vi "General Histogram PtByPt.vi"(0 "x":dbl format="%0.2f", 1 "max":dbl format="%0.2f", 3 "initialize":bool, 5 "Bins":T2(array[cluster]) {"upper" format="%0.2f"; "lower" format="%0.2f"}, 9 "inclusion":enum16{"lower", "upper"}(ring), 11 "sample length":i32=100, 12 "min":dbl format="%0.2f", 14 "# bins":i32) -> (4 "Histogram Graph":T1(graph), 6 "Histogram":i32[](array[numeric]), 8 "Axis":dbl[](array[numeric]), 10 "# outside":cluster{"total":i32, "above":i32, "below":i32}, 15 "error":i32)   [LabVIEW 2020, in "NI_PtbyPt.lvlib"]
doc: "Finds the discrete histogram of the set of input data points specified by <B>sample length</B> based on the given bin specifications."
uses:
  <vilib>/ptbypt/NI_PtbyPt.lvlib
  <vilib>/Analysis/NI_AALPro.lvlib
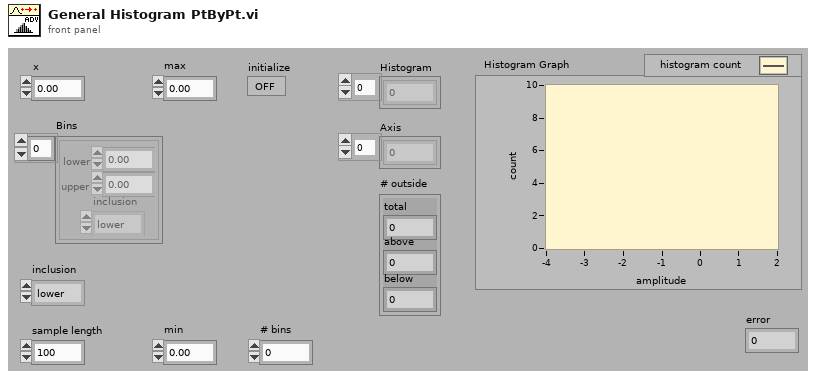
[diagram p1: front panel]
types:
  T1 = cluster{"X Values":dbl[], "Histogram: h(x)":i32[]}
  T2 = cluster{"lower":dbl, "upper":dbl, "inclusion":enum32{"lower", "upper", "both", "neither"}}[]
  T3 = cluster{"lower":dbl, "upper":dbl, "inclusion":u32}[]
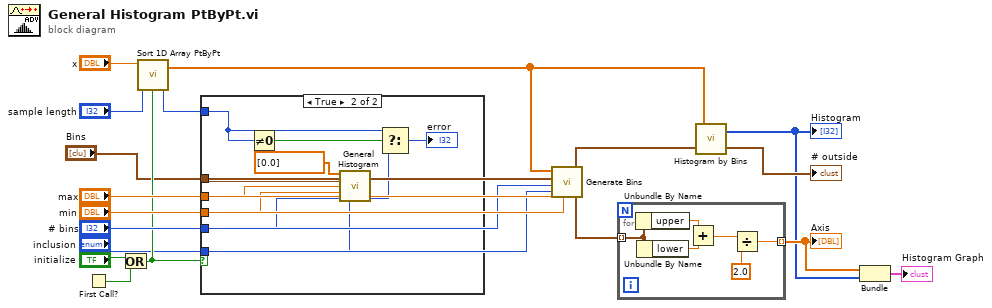
[diagram p0: block diagram]
diagram:
  n1 = First Call?() -> (First Call?: T/F=w7:bool)
  n2 = Or(x="initialize", y=w7) -> (x .or. y?=w9:bool)
  n3 = call <vilib>:"Sort 1D Array PtByPt.vi"("initialize"=w9, "sample length"="sample length", "input data point"="x") -> ("error"=w15:i32, "sorted array"=w10:dbl[])  [unwired: 1 in]
  n4 = case shown="True" w9 {
    tunnel: "Bins" -> [_ w22]
    tunnel: "max" -> [_ w19]
    tunnel: "min" -> [_ w18]
    tunnel: "# bins" -> [_ w21]
    tunnel: "inclusion" -> [_ w20]
    tunnel: w15 -> [_ w25]
    frame False {
    }
    frame True {
      n5 = Not Equal To 0?(x=w25) -> (x != 0?=w26:bool)
      n6 = call <vilib>:"General Histogram.vi"("X"=dbl[] [0.0], "Bins"=w22, "max"=w19, "min"=w18, "# bins"=w21, "inclusion"=w20) -> ("error"=w24:i32)  [unwired: 5 in, 4 out]
      n7 = Select(t=w25, s=w26, f=w24) -> (s? t:f=→"error":i32)
    }
  }
  n8 = call <vilib>:"Generate Bins.vi"("min"="min", "max"="max", "inclusion"="inclusion", "# bins"="# bins", "Bins"="Bins", "Input Data"=w10) -> ("Bins out"=w11:T3)
  n9 = for {
    tunnel: w11 -> [w33] mode=indexing
    tunnel: [w28] -> w3 mode=indexing
    n10 = Unbundle By Name(w33) -> ("upper"=w32:dbl)
    n11 = Unbundle By Name(w33) -> ("lower"=w31:dbl)
    n12 = Add(x=w32, y=w31) -> (x+y=w29:dbl)
    n13 = Divide(x=w29, y=2.0) -> (x/y=w28:dbl)
  }
  "Axis" <- w3
  n14 = call <vilib>:"Histogram by Bins.vi"("Bins"=w11, "Input Data"=w10) -> ("# outside"=→"# outside":cluster{"total":i32, "above":i32, "below":i32}, "Histogram"=w2:i32[])
  "Histogram" <- w2
  n15 = Bundle(w3, "Histogram"=w2) -> (→"Histogram Graph":cluster{dbl[], "Histogram":i32[]})  [unwired: 1 in]
